vi "Write Name.vi"(10 "Name":string, 11 "(Index_Pointer) in":refnum<class "Absolute_Pointer.lvclass">) -> (3 "(Index_Pointer) out":refnum<class "Absolute_Pointer.lvclass">)   [LabVIEW 2024, in "Absolute_Pointer.lvclass"]
uses:
  Absolute_Pointer.lvclass
  _Pointer.lvclass
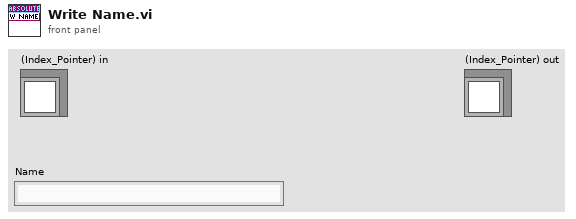
[diagram p1: front panel]
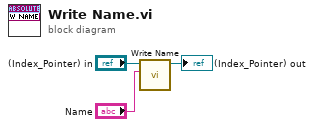
[diagram p0: block diagram]
diagram:
  n1 = call-parent "Write Name.vi"("Name"="Name", "((Pointer)) in"="(Index_Pointer) in") -> ("((Pointer)) out"=→"(Index_Pointer) out":refnum<class "Absolute_Pointer.lvclass">)  [unwired: 9 in]
